vi "Begin.vi"(11 "Image Size":T1=enum."160x120") -> (0 "error out":errorcluster)   [LabVIEW 2012]
doc: "Called before other user functions, this VI is expected to open initial I/O refnums, load in file data, and do all program initialization. Notice that the <B>error out</B> terminal is simply used for data flow. Wiring it to other structures or subVIs ensures that this VI runs first."
uses:
  <vilib>/Rock Robotics/WPI/Camera/WPI_CameraImageSize.ctl
  <vilib>/Rock Robotics/WPI/Camera/WPI_CameraWhite Balance Values.ctl
  <vilib>/Rock Robotics/WPI/Camera/WPI_CameraExposure Values.ctl
  <vilib>/Rock Robotics/WPI/Camera/WPI_CameraFrameRate.ctl
  <vilib>/Rock Robotics/WPI/DriverStation/WPI_DriverStationRobotMode2.ctl
  <vilib>/Rock Robotics/WPI/Relay/WPI_RelayDirection.ctl
  <vilib>/Rock Robotics/SystemInterfaces/DIO/FPGA_DIORelayChannel.ctl
  <vilib>/Rock Robotics/SystemInterfaces/DIO/FPGA_DIOPWMChannel.ctl
  <vilib>/Rock Robotics/SystemInterfaces/Typedef/FPGA_TypedefDigitalModule.ctl
  <vilib>/Rock Robotics/WPI/Joystick/WPI_JoystickDeviceEnum.ctl
  <vilib>/Rock Robotics/SystemInterfaces/DIO/FPGA_DIOChannel.ctl
  <vilib>/Rock Robotics/SystemInterfaces/AI/FPGA_AIGyroChannel.ctl
  <vilib>/Rock Robotics/SystemInterfaces/AI/FPGA_AIChannel.ctl
  Robot Global Data.vi
  <vilib>/Rock Robotics/WPI/MotorControl/WPI_MotorControlOpen Victor.vi
  <vilib>/Rock Robotics/WPI/MotorControl/WPI_MotorControlOpen Jaguar.vi
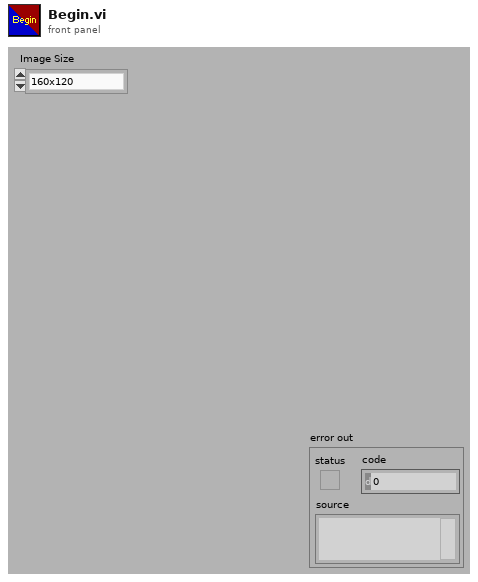
[diagram p1: front panel]
types:
  T1 = typedef "WPI_CameraImageSize.ctl" = enum16{"640x480", "320x240", "160x120"}
  T2 = typedef "FPGA_TypedefDigitalModule.ctl" = enum16{"Digital Module 1", "Digital Module 2"}
  T3 = typedef "FPGA_DIOPWMChannel.ctl" = enum8{"PWM 1", "PWM 2", "PWM 3", "PWM 4", "PWM 5", "PWM 6", "PWM 7", "PWM 8", "PWM 9", "PWM 10", "Invalid"}
  T4 = typedef "WPI_JoystickDeviceEnum.ctl" = enum16{"USB 1", "USB 2", "USB 3", "USB 4", "Kinect 1", "Kinect 2"}
  T5 = typedef "FPGA_DIORelayChannel.ctl" = enum8{"Relay 1", "Relay 2", "Relay 3", "Relay 4", "Relay 5", "Relay 6", "Relay 7", "Relay 8", "Invalid"}
  T6 = typedef "WPI_RelayDirection.ctl" = enum16{"Both directions", "Forward only", "Reverse only"}
  T7 = typedef "WPI_DriverStationRobotMode2.ctl" = enum16{"Autonomous Disabled", "Autonomous Enabled", "Teleop Disabled", "Teleop Enabled", "Timeout", "Finish", "Test Disabled", "Test Enabled"}
  T8 = typedef "WPI_CameraFrameRate.ctl" = u32
  T9 = typedef "WPI_CameraExposure Values.ctl" = enum16{"Auto", "Flicker-free 50 Hz", "Flicker-free 60 Hz", "Hold current"}
  T10 = typedef "WPI_CameraWhite Balance Values.ctl" = enum16{"Auto", "Fixed indoor", "Fixed outdoor 1", "Fixed outdoor 2", "Fixed fluorescent 1", "Fixed fluorescent 2", "Hold current"}
  T11 = typedef "WPI_ServoDeviceRef.ctl" = cluster{"DeviceStatus":errorcluster, "Digital Module":T2, "PWM Channel":T3, "DeadBand":T12}
  T12 = typedef "WPI_PWMDeadband.ctl" = cluster{"Name":string, "maxPositivePwm":i32, "minPositivePwm":i32, "centerPwm":i32, "maxNegativePwm":i32, "minNegativePwm":i32, "angularRange":u16}
  T13 = typedef "WPI_CameraDevRef.ctl" = cluster{"Camera Address":string, "CameraStatus":errorcluster, "Acquire Image Notifier":refnum<notifier>}
  T14 = typedef "WPI_MotorControlDeviceRef.ctl" = cluster{"DeviceStatus":errorcluster, "Type":enum16{"PWM", "CAN"}, "PWM":cluster{"Digital Module":T2, "PWM Channel":T3, "DeadBand":T12}, "CAN":cluster{"Device Number":u8, "Control Mode":T15, "Semaphore":T16, "Max Vout":dbl}, "Invert":bool, "TransformRef":T17, "InvTransformRef":T17}
  T15 = typedef "WPI_CANJaguar_ControlMode.ctl" = enum8{"Percent VBus", "Current", "Speed", "Position", "Voltage"}
  T16 = typedef "Semaphore RefNum" = refnum<k1>
  T17 = typedef "WPI_PWMTransform_ConPane.ctl" = refnum<vi>
  T18 = typedef "WPI_JoystickDevRef.ctl" = cluster{"Device":T4}
  T19 = typedef "WPI_RelayDevRef.ctl" = cluster{"DevStatus":errorcluster, "Relay Channel":T5, "Digital Module":T2, "Relay Direction":T6}
  T20 = typedef "FPGA_AIGyroChannel.ctl" = enum8{"AI 1", "AI 2", "Invalid"}
  T21 = typedef "FPGA_DIOChannel.ctl" = enum8{"DIO 1", "DIO 2", "DIO 3", "DIO 4", "DIO 5", "DIO 6", "DIO 7", "DIO 8", "DIO 9", "DIO 10", "DIO 11", "DIO 12", "DIO 13", "DIO 14", "Invalid"}
  T22 = typedef "FPGA_AIChannel.ctl" = enum8{"AI 1", "AI 2", "AI 3", "AI 4", "AI 5", "AI 6", "AI 7", "AI 8", "Invalid"}
  T23 = typedef "WPI_AnalogChannelDevRef.ctl" = cluster{"DevStatus":errorcluster, "Analog Module":T24, "Analog Channel":T22}
  T24 = typedef "FPGA_TypedefAnalogModule.ctl" = enum16{"Analog Module 1", "Analog Module 2"}
  T25 = typedef "WPI_DigitalInputDevRef.ctl" = cluster{"DevStatus":errorcluster, "DIO Channel":T21, "Digital Module":T2}
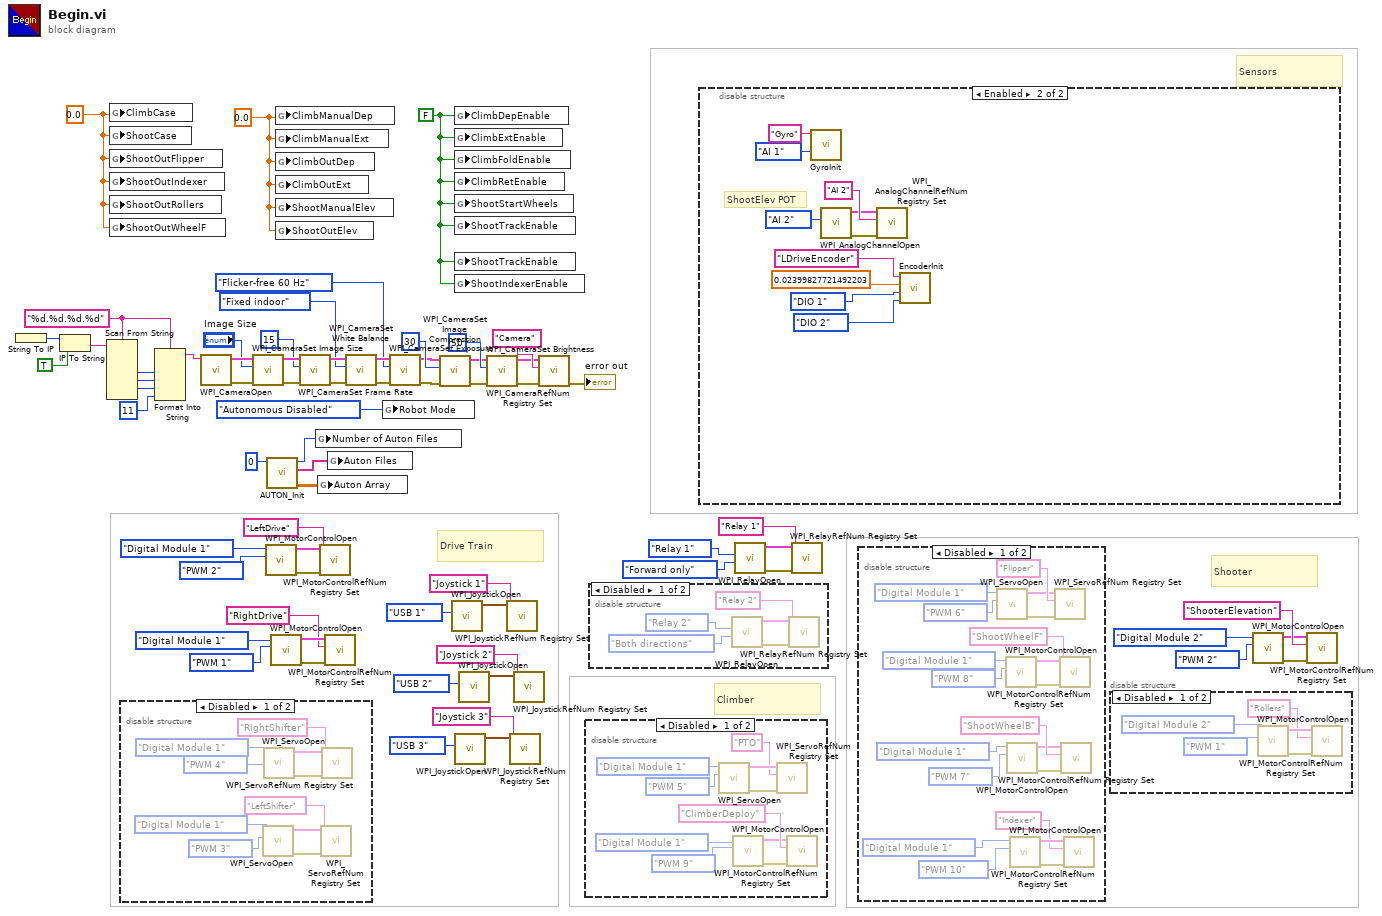
[diagram p0: block diagram]
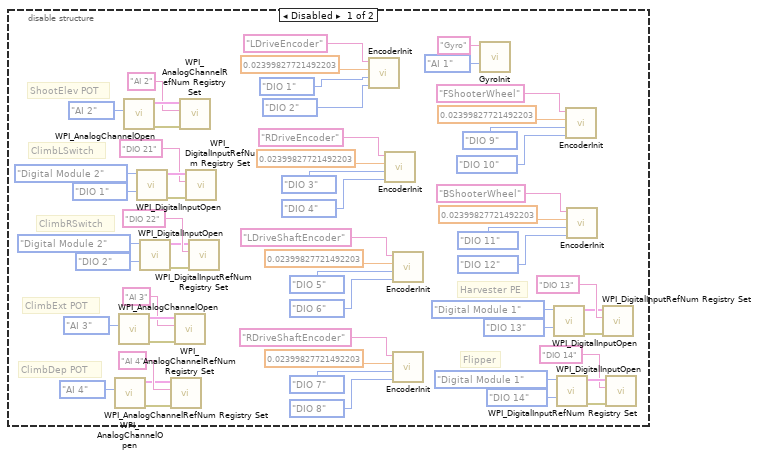
[diagram p6: hidden frame]
diagram:
  w1 = FALSE ("ClimbDepEnable")
  w2 = 0.0 ("ClimbCase")
  w3 = 0.0 ("ClimbCase")
  w40 = "%d.%d.%d.%d" ("format string")
  # "Drive Train"
  # "Climber"
  # "Shooter"
  # "Sensors"
  n1 = String To IP() -> (0:w47:u32)  [unwired: 1 in]
  n2 = IP To String(1:TRUE ("dot notation? (F)"), 2:w47) -> (0:w45:string)
  n3 = Scan From String(format string=w40, input string=w45) -> (output 1=w44:i32, output 2=w43:i32, output 3=w42:i32)  [unwired: 7 in, 3 out]
  n4 = global write "Robot Global Data.vi" "ClimbCase"(w3) -> ()
  n5 = global write "Robot Global Data.vi" "ShootCase"(w3) -> ()
  n6 = global write "Robot Global Data.vi" "ShootOutFlipper"(w3) -> ()
  n7 = global write "Robot Global Data.vi" "ShootOutIndexer"(w3) -> ()
  n8 = global write "Robot Global Data.vi" "ShootOutRollers"(w3) -> ()
  n9 = global write "Robot Global Data.vi" "ShootOutWheelF"(w3) -> ()
  n10 = disable-structure shown="Disabled" {
    frame Disabled {
      n11 = call <vilib>:"WPI_ServoOpen.vi"("PWM Channel"=FPGA_DIOPWMChannel."PWM 3", "Digital Module (Module 1)"=FPGA_TypedefDigitalModule."Digital Module 1") -> ("error out"=w69:errorcluster, "ServoDeviceRef"=w76:T11)  [unwired: 8 in]
      n12 = call <vilib>:"WPI_ServoOpen.vi"("PWM Channel"=FPGA_DIOPWMChannel."PWM 4", "Digital Module (Module 1)"=FPGA_TypedefDigitalModule."Digital Module 1") -> ("error out"=w70:errorcluster, "ServoDeviceRef"=w71:T11)  [unwired: 8 in]
      n13 = call <vilib>:"WPI_ServoRefNum Registry Set.vi"("error in (no error)"=w69, "refnum name"="LeftShifter", "ServoDeviceRef"=w76) -> ()  [unwired: 7 in, 2 out]
      n14 = call <vilib>:"WPI_ServoRefNum Registry Set.vi"("error in (no error)"=w70, "refnum name"="RightShifter", "ServoDeviceRef"=w71) -> ()  [unwired: 7 in, 2 out]
    }
    frame Enabled {
    }
  }
  n15 = Format Into String(format string=w40, w44, w43, w42, 11 ("Compression")) -> (resulting string=w38:string)  [unwired: 2 in, 1 out]
  n16 = call <vilib>:"WPI_CameraOpen.vi"("Camera Address"=w38) -> ("error out"=w59:errorcluster, "CameraDevRef"=w60:T13)  [unwired: 1 in, 8 out]
  n17 = call <vilib>:"WPI_CameraSet Image Size.vi"("error in (no error)"=w59, "Image Size"="Image Size", "CameraDevRef"=w60) -> ("error out"=w58:errorcluster, "CameraDevRef Out"=w61:T13)  [unwired: 7 out]
  n18 = call-poly <vilib>:"WPI_MotorControlOpen.vi"("PWM Channel"=FPGA_DIOPWMChannel."PWM 2", "Digital Module (Module 1)"=FPGA_TypedefDigitalModule."Digital Module 1") -> ("error out"=w18:errorcluster, "MotorControlDeviceRef"=w19:T14)  [unwired: 8 in]
  n19 = call "AUTON_Init.vi"("Default File"=0) -> ("Auton Array"=w33:dbl[][], "Auton Files"=w34:string[], "Number of Auton Files"=w35:i64)  [unwired: 8 in]
  n20 = call-poly <vilib>:"WPI_MotorControlOpen.vi"("PWM Channel"=FPGA_DIOPWMChannel."PWM 1", "Digital Module (Module 1)"=FPGA_TypedefDigitalModule."Digital Module 1") -> ("error out"=w25:errorcluster, "MotorControlDeviceRef"=w24:T14)  [unwired: 8 in]
  n21 = global write "Robot Global Data.vi" "ClimbManualDep"(w2) -> ()
  n22 = global write "Robot Global Data.vi" "ClimbManualExt"(w2) -> ()
  n23 = global write "Robot Global Data.vi" "ClimbOutDep"(w2) -> ()
  n24 = global write "Robot Global Data.vi" "ClimbOutExt"(w2) -> ()
  n25 = global write "Robot Global Data.vi" "ShootManualElev"(w2) -> ()
  n26 = global write "Robot Global Data.vi" "ShootOutElev"(w2) -> ()
  n27 = call <vilib>:"WPI_CameraSet Frame Rate.vi"("error in (no error)"=w58, "Frame Rate (fps)"=T8 15, "CameraDevRef"=w61) -> ("error out"=w57:errorcluster, "CameraDevRef Out"=w63:T13)  [unwired: 7 out]
  n28 = global write "Robot Global Data.vi" "Number of Auton Files"(w35) -> ()
  n29 = global write "Robot Global Data.vi" "Auton Array"(w33) -> ()
  n30 = call <vilib>:"WPI_MotorControlRefNum Registry Set.vi"("error in (no error)"=w18, "refnum name"="LeftDrive", "MotorControlDevRef"=w19) -> ()  [unwired: 7 in, 2 out]
  n31 = call <vilib>:"WPI_MotorControlRefNum Registry Set.vi"("error in (no error)"=w25, "refnum name"="RightDrive", "MotorControlDevRef"=w24) -> ()  [unwired: 7 in, 2 out]
  n32 = global write "Robot Global Data.vi" "Auton Files"(w34) -> ()
  n33 = call <vilib>:"WPI_CameraSet White Balance.vi"("error in (no error)"=w57, "White Balance"=WPI_CameraWhite_Balance_Values."Fixed indoor", "CameraDevRef"=w63) -> ("error out"=w56:errorcluster, "CameraDevRef Out"=w62:T13)  [unwired: 7 out]
  n34 = global write "Robot Global Data.vi" "Robot Mode"(WPI_DriverStationRobotMode2."Autonomous Disabled" ("Robot Mode")) -> ()
  n35 = call <vilib>:"WPI_CameraSet Exposure.vi"("error in (no error)"=w56, "Exposure"=WPI_CameraExposure_Values."Flicker-free 60 Hz", "CameraDevRef"=w62) -> ("error out"=w55:errorcluster, "CameraDevRef Out"=w65:T13)  [unwired: 7 out]
  n36 = call <vilib>:"WPI_CameraSet Image Compression.vi"("error in (no error)"=w55, "Compression"=30, "CameraDevRef"=w65) -> ("error out"=w54:errorcluster, "CameraDevRef Out"=w64:T13)  [unwired: 7 out]
  n37 = call <vilib>:"WPI_JoystickOpen.vi"("JoystickDevice"=WPI_JoystickDeviceEnum."USB 1") -> ("JoystickDevRef"=w9:T18)  [unwired: 10 in]
  n38 = global write "Robot Global Data.vi" "ClimbDepEnable"(w1) -> ()
  n39 = global write "Robot Global Data.vi" "ClimbExtEnable"(w1) -> ()
  n40 = global write "Robot Global Data.vi" "ClimbFoldEnable"(w1) -> ()
  n41 = global write "Robot Global Data.vi" "ClimbRetEnable"(w1) -> ()
  n42 = global write "Robot Global Data.vi" "ShootStartWheels"(w1) -> ()
  n43 = global write "Robot Global Data.vi" "ShootTrackEnable"(w1) -> ()
  n44 = global write "Robot Global Data.vi" "ShootTrackEnable"(w1) -> ()
  n45 = global write "Robot Global Data.vi" "ShootIndexerEnable"(w1) -> ()
  n46 = call <vilib>:"WPI_JoystickOpen.vi"("JoystickDevice"=WPI_JoystickDeviceEnum."USB 3") -> ("JoystickDevRef"=w15:T18)  [unwired: 10 in]
  n47 = call <vilib>:"WPI_JoystickOpen.vi"("JoystickDevice"=WPI_JoystickDeviceEnum."USB 2") -> ("JoystickDevRef"=w14:T18)  [unwired: 10 in]
  n48 = call <vilib>:"WPI_CameraSet Brightness.vi"("error in (no error)"=w54, "Brightness"=50, "CameraDevRef"=w64) -> ("error out"=w52:errorcluster, "CameraDevRef Out"=w53:T13)  [unwired: 7 out]
  n49 = call <vilib>:"WPI_JoystickRefNum Registry Set.vi"("refnum name"="Joystick 1", "JoystickDevRef"=w9) -> ()  [unwired: 8 in, 2 out]
  n50 = call <vilib>:"WPI_JoystickRefNum Registry Set.vi"("refnum name"="Joystick 3", "JoystickDevRef"=w15) -> ()  [unwired: 8 in, 2 out]
  n51 = call <vilib>:"WPI_JoystickRefNum Registry Set.vi"("refnum name"="Joystick 2", "JoystickDevRef"=w14) -> ()  [unwired: 8 in, 2 out]
  n52 = call <vilib>:"WPI_CameraRefNum Registry Set.vi"("error in (no error)"=w52, "refnum name"="Camera", "CameraDevRef"=w53) -> ("error out"=→"error out":errorcluster)  [unwired: 8 out]
  n53 = disable-structure shown="Disabled" {
    frame Disabled {
      n54 = call <vilib>:"WPI_ServoOpen.vi"("PWM Channel"=FPGA_DIOPWMChannel."PWM 5", "Digital Module (Module 1)"=FPGA_TypedefDigitalModule."Digital Module 1") -> ("error out"=w88:errorcluster, "ServoDeviceRef"=w87:T11)  [unwired: 8 in]
      n55 = call-poly <vilib>:"WPI_MotorControlOpen.vi"("PWM Channel"=FPGA_DIOPWMChannel."PWM 9", "Digital Module (Module 1)"=FPGA_TypedefDigitalModule."Digital Module 1") -> ("error out"=w82:errorcluster, "MotorControlDeviceRef"=w81:T14)  [unwired: 8 in]
      n56 = call <vilib>:"WPI_ServoRefNum Registry Set.vi"("error in (no error)"=w88, "refnum name"="PTO", "ServoDeviceRef"=w87) -> ()  [unwired: 7 in, 2 out]
      n57 = call <vilib>:"WPI_MotorControlRefNum Registry Set.vi"("error in (no error)"=w82, "refnum name"="ClimberDeploy", "MotorControlDevRef"=w81) -> ()  [unwired: 7 in, 2 out]
    }
    frame Enabled {
    }
  }
  n58 = disable-structure shown="Disabled" {
    frame Disabled {
      n59 = call <vilib>:"WPI_RelayOpen.vi"("Relay Direction"=WPI_RelayDirection."Both directions", "Relay Channel"=FPGA_DIORelayChannel."Relay 2") -> ("error out"=w89:errorcluster, "RelayDevRef"=w90:T19)  [unwired: 8 in]
      n60 = call <vilib>:"WPI_RelayRefNum Registry Set.vi"("error in (no error)"=w89, "refnum name"="Relay 2", "RelayDevRef"=w90) -> ()  [unwired: 7 in, 2 out]
    }
    frame Enabled {
    }
  }
  n61 = disable-structure shown="Enabled" {
    frame Disabled {
      # "ShootElev POT"
      # "ClimbRSwitch"
      # "ClimbLSwitch"
      # "ClimbDep POT"
      # "ClimbExt POT"
      # "Flipper"
      # "Harvester PE"
      n62 = call <vilib>:"WPI_AnalogChannelOpen.vi"("Analog Channel"=FPGA_AIChannel."AI 4") -> ("error out"=w118:errorcluster, "AIDeviceRef"=w119:T23)  [unwired: 9 in]
      n63 = call <vilib>:"WPI_AnalogChannelOpen.vi"("Analog Channel"=FPGA_AIChannel."AI 3") -> ("error out"=w117:errorcluster, "AIDeviceRef"=w116:T23)  [unwired: 9 in]
      n64 = call <vilib>:"WPI_AnalogChannelOpen.vi"("Analog Channel"=FPGA_AIChannel."AI 2") -> ("error out"=w100:errorcluster, "AIDeviceRef"=w102:T23)  [unwired: 9 in]
      n65 = call <vilib>:"WPI_DigitalInputOpen.vi"("DIO Channel"=FPGA_DIOChannel."DIO 1", "Digital Module (Module 1)"=FPGA_TypedefDigitalModule."Digital Module 2") -> ("error out"=w105:errorcluster, "DigitalInputDevRef"=w106:T25)  [unwired: 8 in]
      n66 = call <vilib>:"WPI_DigitalInputOpen.vi"("DIO Channel"=FPGA_DIOChannel."DIO 2", "Digital Module (Module 1)"=FPGA_TypedefDigitalModule."Digital Module 2") -> ("error out"=w112:errorcluster, "DigitalInputDevRef"=w111:T25)  [unwired: 8 in]
      n67 = call <vilib>:"WPI_AnalogChannelRefNum Registry Set.vi"("error in (no error)"=w118, "refnum name"="AI 4", "AIDeviceRef"=w119) -> ()  [unwired: 7 in, 2 out]
      n68 = call <vilib>:"WPI_AnalogChannelRefNum Registry Set.vi"("error in (no error)"=w117, "refnum name"="AI 3", "AIDeviceRef"=w116) -> ()  [unwired: 7 in, 2 out]
      n69 = call <vilib>:"WPI_AnalogChannelRefNum Registry Set.vi"("error in (no error)"=w100, "refnum name"="AI 2", "AIDeviceRef"=w102) -> ()  [unwired: 7 in, 2 out]
      n70 = call <vilib>:"WPI_DigitalInputRefNum Registry Set.vi"("error in (no error)"=w105, "refnum name"="DIO 21", "DigitalInputDevRef"=w106) -> ()  [unwired: 7 in, 2 out]
      n71 = call <vilib>:"WPI_DigitalInputRefNum Registry Set.vi"("error in (no error)"=w112, "refnum name"="DIO 22", "DigitalInputDevRef"=w111) -> ()  [unwired: 7 in, 2 out]
      n72 = call "EncoderInit.vi"("refnum name"="LDriveEncoder", "DistancePerCount"=0.02399827721492203, "DIO Channel"=FPGA_DIOChannel."DIO 1", "DIO Channel 2"=FPGA_DIOChannel."DIO 2") -> ()  [unwired: 7 in]
      n73 = call "EncoderInit.vi"("refnum name"="RDriveEncoder", "DistancePerCount"=0.02399827721492203, "DIO Channel"=FPGA_DIOChannel."DIO 3", "DIO Channel 2"=FPGA_DIOChannel."DIO 4") -> ()  [unwired: 7 in]
      n74 = call "EncoderInit.vi"("refnum name"="LDriveShaftEncoder", "DistancePerCount"=0.02399827721492203, "DIO Channel"=FPGA_DIOChannel."DIO 5", "DIO Channel 2"=FPGA_DIOChannel."DIO 6") -> ()  [unwired: 7 in]
      n75 = call "EncoderInit.vi"("refnum name"="RDriveShaftEncoder", "DistancePerCount"=0.02399827721492203, "DIO Channel"=FPGA_DIOChannel."DIO 7", "DIO Channel 2"=FPGA_DIOChannel."DIO 8") -> ()  [unwired: 7 in]
      n76 = call "GyroInit.vi"("refnum name"="Gyro", "Analog Channel"=FPGA_AIGyroChannel."AI 1") -> ()  [unwired: 8 in]
      n77 = call <vilib>:"WPI_DigitalInputOpen.vi"("DIO Channel"=FPGA_DIOChannel."DIO 13", "Digital Module (Module 1)"=FPGA_TypedefDigitalModule."Digital Module 1") -> ("error out"=w130:errorcluster, "DigitalInputDevRef"=w129:T25)  [unwired: 8 in]
      n78 = call <vilib>:"WPI_DigitalInputOpen.vi"("DIO Channel"=FPGA_DIOChannel."DIO 14", "Digital Module (Module 1)"=FPGA_TypedefDigitalModule."Digital Module 1") -> ("error out"=w123:errorcluster, "DigitalInputDevRef"=w124:T25)  [unwired: 8 in]
      n79 = call "EncoderInit.vi"("refnum name"="FShooterWheel", "DistancePerCount"=0.02399827721492203, "DIO Channel"=FPGA_DIOChannel."DIO 9", "DIO Channel 2"=FPGA_DIOChannel."DIO 10") -> ()  [unwired: 7 in]
      n80 = call "EncoderInit.vi"("refnum name"="BShooterWheel", "DistancePerCount"=0.02399827721492203, "DIO Channel"=FPGA_DIOChannel."DIO 11", "DIO Channel 2"=FPGA_DIOChannel."DIO 12") -> ()  [unwired: 7 in]
      n81 = call <vilib>:"WPI_DigitalInputRefNum Registry Set.vi"("error in (no error)"=w130, "refnum name"="DIO 13", "DigitalInputDevRef"=w129) -> ()  [unwired: 7 in, 2 out]
      n82 = call <vilib>:"WPI_DigitalInputRefNum Registry Set.vi"("error in (no error)"=w123, "refnum name"="DIO 14", "DigitalInputDevRef"=w124) -> ()  [unwired: 7 in, 2 out]
    }
    frame Enabled {
      # "ShootElev POT"
      n83 = call "GyroInit.vi"("refnum name"="Gyro", "Analog Channel"=FPGA_AIGyroChannel."AI 1") -> ()  [unwired: 8 in]
      n84 = call <vilib>:"WPI_AnalogChannelOpen.vi"("Analog Channel"=FPGA_AIChannel."AI 2") -> ("error out"=w161:errorcluster, "AIDeviceRef"=w158:T23)  [unwired: 9 in]
      n85 = call <vilib>:"WPI_AnalogChannelRefNum Registry Set.vi"("error in (no error)"=w161, "refnum name"="AI 2", "AIDeviceRef"=w158) -> ()  [unwired: 7 in, 2 out]
      n86 = call "EncoderInit.vi"("refnum name"="LDriveEncoder", "DistancePerCount"=0.02399827721492203, "DIO Channel"=FPGA_DIOChannel."DIO 1", "DIO Channel 2"=FPGA_DIOChannel."DIO 2") -> ()  [unwired: 7 in]
    }
  }
  n87 = call <vilib>:"WPI_RelayOpen.vi"("Relay Direction"=WPI_RelayDirection."Forward only", "Relay Channel"=FPGA_DIORelayChannel."Relay 1") -> ("error out"=w32:errorcluster, "RelayDevRef"=w31:T19)  [unwired: 8 in]
  n88 = call <vilib>:"WPI_RelayRefNum Registry Set.vi"("error in (no error)"=w32, "refnum name"="Relay 1", "RelayDevRef"=w31) -> ()  [unwired: 7 in, 2 out]
  n89 = disable-structure shown="Disabled" {
    frame Disabled {
      n90 = call <vilib>:"WPI_ServoOpen.vi"("PWM Channel"=FPGA_DIOPWMChannel."PWM 6", "Digital Module (Module 1)"=FPGA_TypedefDigitalModule."Digital Module 1") -> ("error out"=w167:errorcluster, "ServoDeviceRef"=w168:T11)  [unwired: 8 in]
      n91 = call-poly <vilib>:"WPI_MotorControlOpen.vi"("PWM Channel"=FPGA_DIOPWMChannel."PWM 8", "Digital Module (Module 1)"=FPGA_TypedefDigitalModule."Digital Module 1") -> ("error out"=w178:errorcluster, "MotorControlDeviceRef"=w179:T14)  [unwired: 8 in]
      n92 = call-poly <vilib>:"WPI_MotorControlOpen.vi"("PWM Channel"=FPGA_DIOPWMChannel."PWM 7", "Digital Module (Module 1)"=FPGA_TypedefDigitalModule."Digital Module 1") -> ("error out"=w164:errorcluster, "MotorControlDeviceRef"=w163:T14)  [unwired: 8 in]
      n93 = call-poly <vilib>:"WPI_MotorControlOpen.vi"("PWM Channel"=FPGA_DIOPWMChannel."PWM 10", "Digital Module (Module 1)"=FPGA_TypedefDigitalModule."Digital Module 1") -> ("error out"=w174:errorcluster, "MotorControlDeviceRef"=w175:T14)  [unwired: 8 in]
      n94 = call <vilib>:"WPI_ServoRefNum Registry Set.vi"("error in (no error)"=w167, "refnum name"="Flipper", "ServoDeviceRef"=w168) -> ()  [unwired: 7 in, 2 out]
      n95 = call <vilib>:"WPI_MotorControlRefNum Registry Set.vi"("error in (no error)"=w178, "refnum name"="ShootWheelF", "MotorControlDevRef"=w179) -> ()  [unwired: 7 in, 2 out]
      n96 = call <vilib>:"WPI_MotorControlRefNum Registry Set.vi"("error in (no error)"=w164, "refnum name"="ShootWheelB", "MotorControlDevRef"=w163) -> ()  [unwired: 7 in, 2 out]
      n97 = call <vilib>:"WPI_MotorControlRefNum Registry Set.vi"("error in (no error)"=w174, "refnum name"="Indexer", "MotorControlDevRef"=w175) -> ()  [unwired: 7 in, 2 out]
    }
    frame Enabled {
    }
  }
  n98 = disable-structure shown="Disabled" {
    frame Disabled {
      n99 = call-poly <vilib>:"WPI_MotorControlOpen.vi"("PWM Channel"=FPGA_DIOPWMChannel."PWM 1", "Digital Module (Module 1)"=FPGA_TypedefDigitalModule."Digital Module 2") -> ("error out"=w184:errorcluster, "MotorControlDeviceRef"=w185:T14)  [unwired: 8 in]
      n100 = call <vilib>:"WPI_MotorControlRefNum Registry Set.vi"("error in (no error)"=w184, "refnum name"="Rollers", "MotorControlDevRef"=w185) -> ()  [unwired: 7 in, 2 out]
    }
    frame Enabled {
    }
  }
  n101 = call-poly <vilib>:"WPI_MotorControlOpen.vi"("PWM Channel"=FPGA_DIOPWMChannel."PWM 2", "Digital Module (Module 1)"=FPGA_TypedefDigitalModule."Digital Module 2") -> ("error out"=w6:errorcluster, "MotorControlDeviceRef"=w5:T14)  [unwired: 8 in]
  n102 = call <vilib>:"WPI_MotorControlRefNum Registry Set.vi"("error in (no error)"=w6, "refnum name"="ShooterElevation", "MotorControlDevRef"=w5) -> ()  [unwired: 7 in, 2 out]
